vi "B-Scan.vi"(7 "Micropulse # In":i32, 9 "Scan definition":T1={"Scan Start"=0.0, "Scan Length"=280.0, "Inspection Resolution"=0.5, "Direction"=enum."Forwards"} {"Inspection Resolution" format="%#_6f"; "Scan Start" format="%#_6f"; "Scan Length" format="%#_6f"}, 11 "scan data info":T3 {"Error Message" format="%04x"; "Message Header" format="%04x"; "IP"."MIP location" format="%#.0f"; "IP"."Location" format="%#.0f"; "PRF" format="%.0fHz"}) -> (2 "B-Scan Out":u16[][](array[numeric]))   [LabVIEW 2026, in "MicroPulse_Driver.lvlib"]
uses:
  MicroPulse_Driver.lvlib
  Data/Datatypes/MP - data output format.ctl
  <instrlib>/Micropulse/Micropulse.lvlib
  Data/Datatypes/MP - retain scan.ctl
  Data/Datatypes/MP - scan data info.ctl
  Data/Datatypes/MP - inspection direction.ctl
  Data/Datatypes/MP - fly scan range.ctl
  Data/Datatypes/MP - axis positions (LLC).ctl
panel:
  out "Update Display?":bool
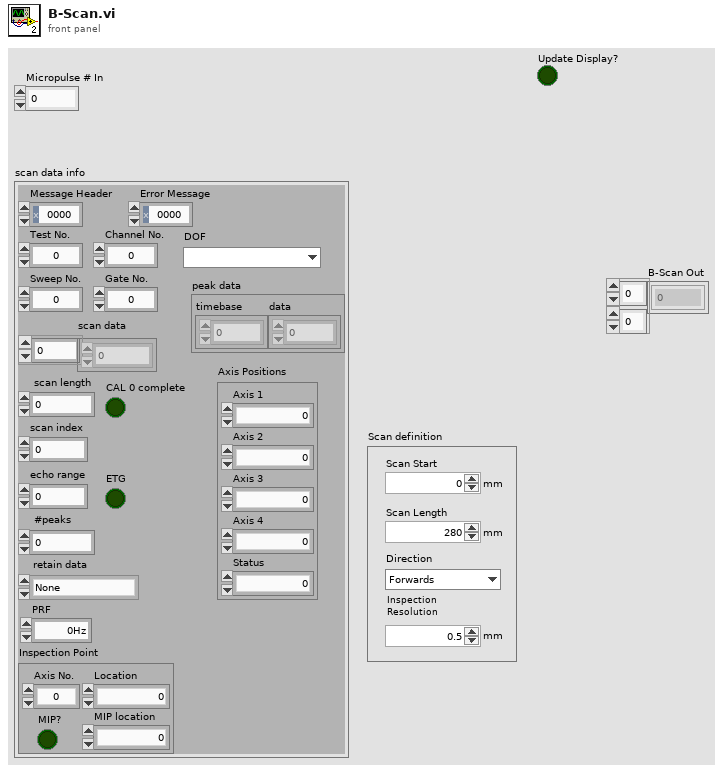
[diagram p1: front panel]
types:
  T1 = typedef "Micropulse.lvlib/MP - fly scan range.ctl" = cluster{"Scan Start":dbl, "Scan Length":dbl, "Inspection Resolution":dbl, "Direction":T2}
  T2 = typedef "Micropulse.lvlib/MP - inspection direction.ctl" = enum16{"Forwards", "Backwards"}
  T3 = typedef "Micropulse.lvlib/MP - scan data info.ctl" = cluster{"Message Header":u16, "Error Message":u16, "Test No.":u32, "Channel No.":u8, "Sweep No.":u32, "Gate No.":u32, "DOF":T4, "retain data":T5, "scan data":u16[], "scan length":i32, "scan index":i32, "peak data":cluster{"timebase":u16[], "data":u16[]}, "#peaks":i32, "PRF":dbl, "IP":cluster{"Axis No.":u8, "Location":u32, "MIP location":u32, "MIP?":bool}, "echo range":u16, "ETG":bool, "CAL 0 complete":bool, "Axis Positions":T6}
  T4 = typedef "Micropulse.lvlib/MP - data output format.ctl" = enum16{"", "8-bit Mode", "10-bit Mode", "12-bit Mode", "16-bit Mode", "8-bit Log Mode", "12-bit Packed Mode"}
  T5 = typedef "Micropulse.lvlib/MP - retain scan.ctl" = enum16{"None", "Ascan", "Peaks"}
  T6 = typedef "Micropulse.lvlib/MP - axis positions (LLC).ctl" = cluster{"Axis 1":u32, "Axis 2":u32, "Axis 3":u32, "Axis 4":u32, "Status":u8}
  T7 = enum16{"Read", "Start B-Scan", "B-Scan Finished"}
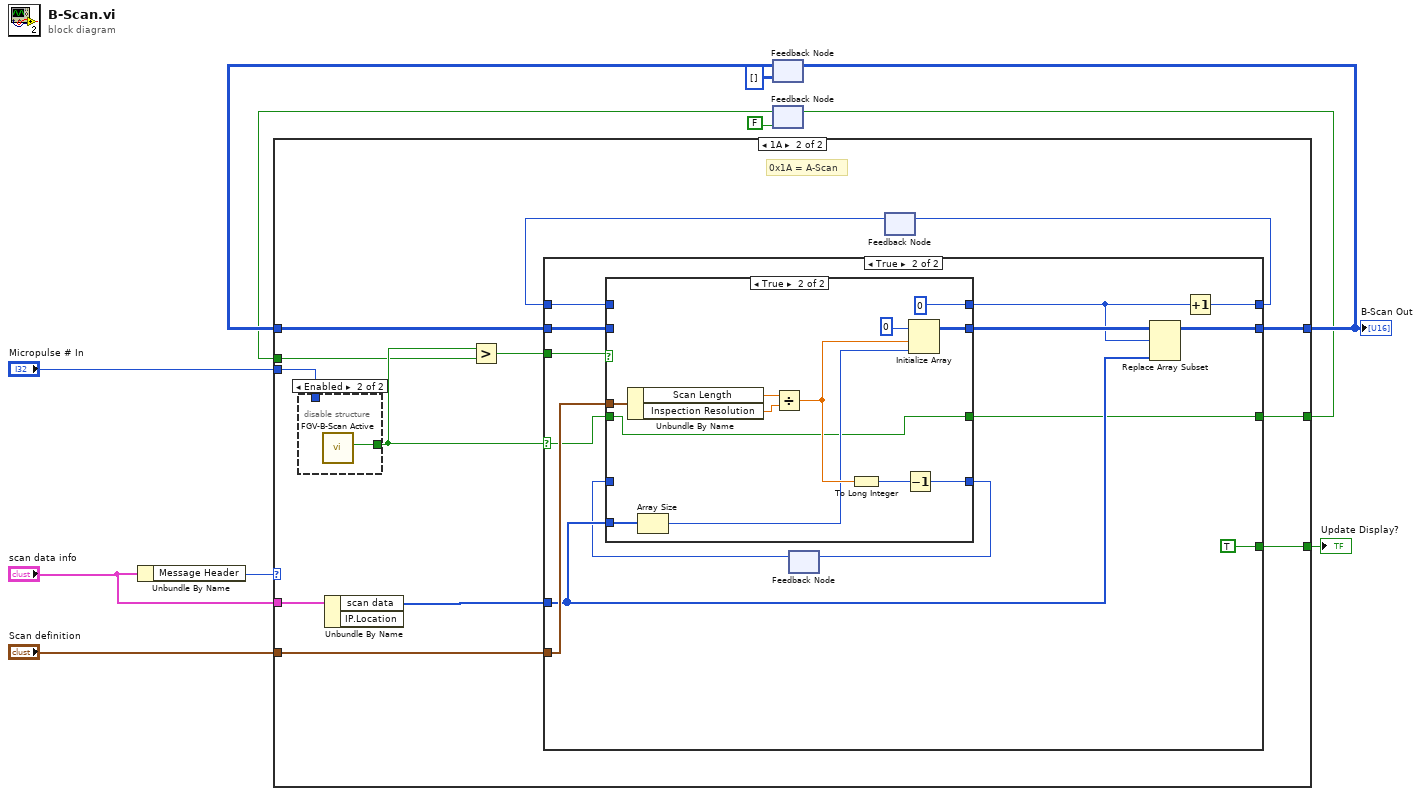
[diagram p0: block diagram]
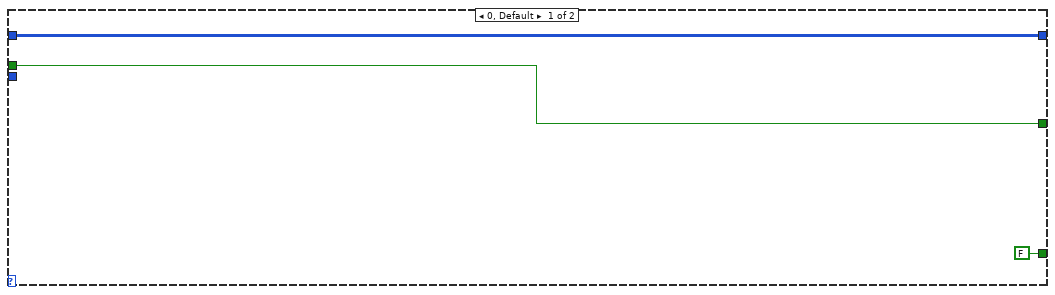
[diagram p2: hidden frame]
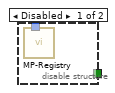
[diagram p3: hidden frame]
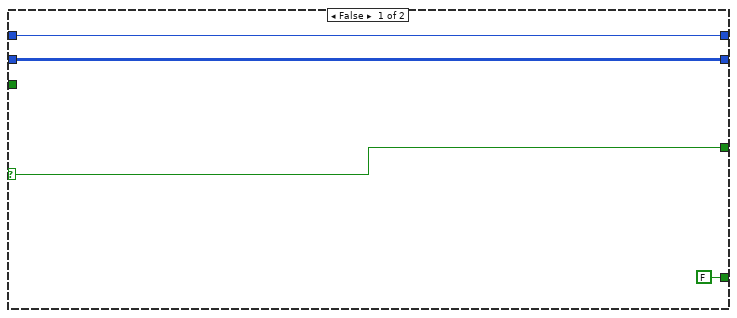
[diagram p4: hidden frame]
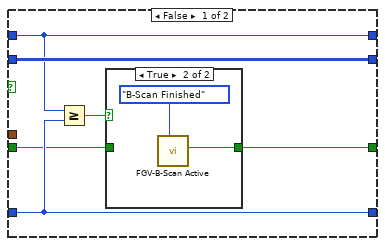
[diagram p5: hidden frame]
diagram:
  n1 = Unbundle By Name("scan data info") -> ("Message Header"=w11:u16)
  n2 = feedback #1(u16[][] []) -> (w7:u16[][])
  n3 = feedback #2(FALSE ("B-Scan In Progress?")) -> (w3:bool)
  n4 = case shown="1A" w11 {
    tunnel: "scan data info" -> [_ w27]
    tunnel: "Scan definition" -> [_ w25]
    tunnel: [w14 w22] -> w8
    tunnel: w7 -> [w14 w21]
    tunnel: "Micropulse # In" -> [_ w20]
    tunnel: [w13 w17] -> w4
    tunnel: w3 -> [w13 w16]
    tunnel: [FALSE w15] -> w1
    frame 0, Default {
    }
    frame 26 {
      # "0x1A = A-Scan"
      n5 = disable-structure shown="Enabled" {
        disable-tunnel: w20 -> [w28 _]
        disable-tunnel: [_ w29] -> w18
        frame Disabled {
          n6 = call "MP-Registry.vi"("Micropulse # In"=w28) -> ()  [unwired: 7 in, 4 out]
        }
        frame Enabled {
          n7 = call "FGV-B-Scan Active.vi"() -> ("B-Scan Start?"=w29:bool)  [unwired: 9 in, 2 out]
        }
      }
      n8 = Unbundle By Name(w27) -> ("scan data"=w26:u16[])  [unwired: 1 out]
      n9 = Greater?(x=w18, y=w16) -> (0:w19:bool)
      n10 = feedback #3() -> (w23:i32)  [unwired: 1 in]
      n11 = case shown="True" w18 {
        selector: w18 -> [w31 w35]
        tunnel: w19 -> [_ w45]
        tunnel: w21 -> [w33 w47]
        tunnel: [w33 w44] -> w22
        tunnel: w26 -> [_ w41]
        tunnel: w25 -> [_ w43]
        tunnel: [w32 w40] -> w24
        tunnel: w23 -> [w32 w42]
        tunnel: [w31 w36] -> w17
        tunnel: [FALSE TRUE] -> w15
        frame False {
        }
        frame True {
          n12 = feedback #4() -> (w38:i32)  [unwired: 1 in]
          n13 = case shown="True" w45 {
            tunnel: w47 -> [w53 _]
            tunnel: [w53 w68] -> w46
            tunnel: w43 -> [_ w66]
            tunnel: w41 -> [_ w63]
            tunnel: [w52 0 ("index")] -> w37
            tunnel: w42 -> [w52 _]
            tunnel: [w51 w61] -> w39
            tunnel: w38 -> [w51 _]
            tunnel: [w49 w57] -> w36
            tunnel: w35 -> [w48 w57]
            frame False {
              n14 = Greater Or Equal?(x=w52, y=w51) -> (x >= y?=w50:bool)
              n15 = case shown="True" w50 {
                tunnel: [w54 w55] -> w49
                tunnel: w48 -> [w54 _]
                frame False {
                }
                frame True {
                  n16 = call "FGV-B-Scan Active.vi"("Action"=T7."B-Scan Finished") -> ("B-Scan Start?"=w55:bool)  [unwired: 8 in, 2 out]
                }
              }
            }
            frame True {
              n17 = Unbundle By Name(w66) -> ("Scan Length"=w65:dbl, "Inspection Resolution"=w64:dbl)
              n18 = Array Size(array=w63) -> (size(s)=w58:i32)
              n19 = Divide(x=w65, y=w64) -> (x/y=w59:dbl)
              n20 = To Long Integer(number=w59) -> (32bit integer=w60:i32)
              n21 = Decrement(x=w60) -> (x-1=w61:i32)
              n22 = Initialize Array(u16 0 ("index"), w59, w58) -> (w68:u16[][])
            }
          }
          n23 = feedback-in #4(w39) -> ()
          n24 = Replace Array Subset(array=w46, new element=w41, index (row)=w37) -> (w44:u16[][])  [unwired: 1 in]
          n25 = Increment(x=w37) -> (x+1=w40:i32)
        }
      }
      n26 = feedback-in #3(w24) -> ()
    }
  }
  "B-Scan Out" <- w8
  "Update Display?" <- w1
  n27 = feedback-in #1(w8) -> ()
  n28 = feedback-in #2(w4) -> ()
